vi "RandSelectSpeed.vi"(11 "Array":dbl[](array[numeric])) -> (3 "Numeric":dbl)   [LabVIEW 2013]
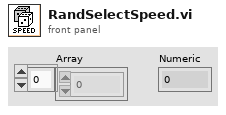
[diagram p1: front panel]
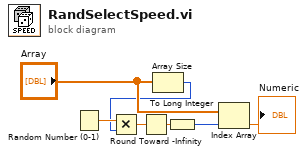
[diagram p0: block diagram]
diagram:
  n1 = Random Number (0-1)() -> (number: 0 to 1=w5:dbl)
  n2 = Array Size(array="Array") -> (size(s)=w1:i32)
  n3 = Multiply(x=w5, y=w1) -> (x*y=w4:dbl)
  n4 = Round Toward -Infinity(1:w4) -> (0:w2:dbl)
  n5 = To Long Integer(number=w2) -> (32bit integer=w3:i32)
  n6 = Index Array(array="Array", index=w3) -> (element=→"Numeric":dbl)
